vi "波形前面板显示.vi"(9 "ORP滴定曲线":u16[](graph), 10 "滴定数-ORP值":u16[](array[numeric]) caption="数组", 11 "波形时间":timestamp) -> ()   [LabVIEW 2016]
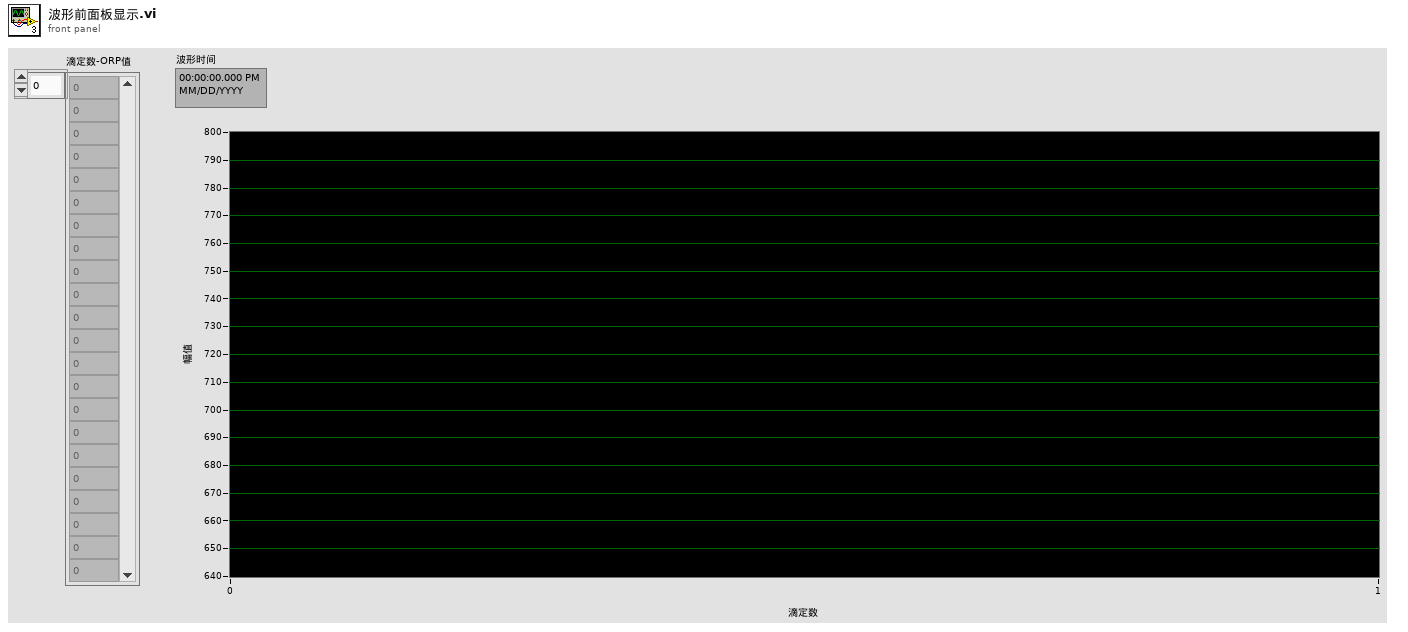
[diagram p1: front panel]
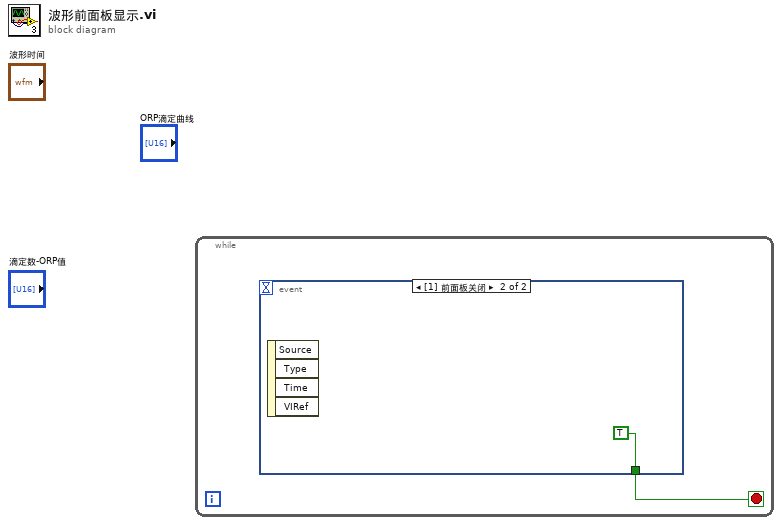
[diagram p0: block diagram]
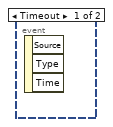
[diagram p2: hidden frame]
diagram:
  n1 = while {
    stop <- w1 stop-if-true
    n2 = event shown="[1] 前面板关闭" {
      selector: _ -> [_ _]
      dyn-events: _ -> [_ _]
      timeout: _ -> [_ _]
      tunnel: [_ TRUE] -> w1
      event Timeout {
        n3 = event-data() -> ()  [unwired: 1 in, 3 out]
      }
      event Panel Close {
        n4 = event-data() -> ()  [unwired: 1 in, 4 out]
      }
    }
  }
